vi "Read_raw_inst_setup.vi"(0 "Setup file":string) -> (8 "Setup string":string, 10 "Ch & spans choices":T4(array[cluster]) {"D" format="%.2f"; "Ch No" min=0; "low limit (-10V)" min=-10 max=10 format="%.2f"; "high limit (10V)" min=-10 max=10 format="%.2f"}, 13 "PWA Data":T1, 14 "Number of Analogue instruments":i32=1, 16 "LDA data":enum16{"No LDA data", "Take LDA data"}(ring)=enum."Take LDA data", 17 "LDA set up":T3={"dimensions"=enum."2D", "Analogue Freq Multiplier"=0.1} {"Analogue Freq Multiplier" min=0.1 max=100.0 format="%_5g"}, 19 "Synchronise Analogue channels with LDA":bool)   [LabVIEW 2014]
uses:
  Controls/Inst_type.ctl
  Controls/LDA_Setup.ctl
  Controls/PWA_Data.ctl
  Controls/Post_Process.ctl
  File/Setup_Filetype.ctl
  Controls/Trigger_Mode.ctl
  Controls/Tunnel_Coordinates.ctl
  Globals/Meas_global.vi
  Globals/LDA_meas_global_1.vi
  Globals/LDA_meas_global_2.vi
  Globals/Trav_pos_global.vi
panel:
  in  "Inst type":T2
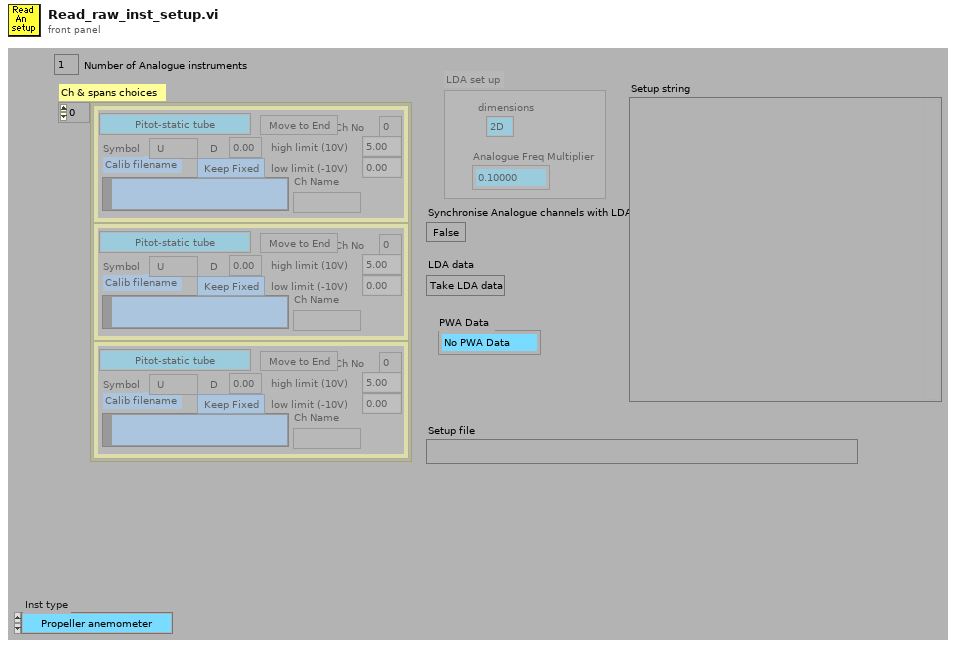
[diagram p1: front panel]
types:
  T1 = typedef "PWA_Data.ctl" = enum16{"No PWA Data", "One Ch PWA"}
  T2 = typedef "Inst_type.ctl" = enum16{"Propeller anemometer", "Raw voltage", "Pressure Transducer", "Pitot-static tube", "Preston tube", "Hot wire", "Cross wire 1", "Cross wire 2", "Generic Linear", "Generic Polynomial", "Generic BackPoly", "Fast FID", "Thermocouple", "Cold wire", "Pulsed Wire", "LDA Vel", "LDA Tran time", "LDA Arr time", "Microphone"}
  T3 = typedef "LDA_Setup.ctl" = cluster{"dimensions":enum16{"1D", "2D"}, "Analogue Freq Multiplier":dbl}
  T4 = cluster{"high limit (10V)":sgl, "low limit (-10V)":sgl, "Ch No":i16, "Calib filename":path, "Inst type":T2, "Symbol":string, "Move channel":bool, "Use Latest":bool, "D":dbl, "Ch Name":string}[]
  T5 = typedef "Post_Process.ctl" = enum16{"Take New Data", "Post Process Raw Data File"}
  T6 = typedef "Setup_Filetype.ctl" = enum16{"Measurement Setups", "Calibration Setups", "General", "Results File Plotter Setups", "Speed Calib Tweaks"}
  T7 = typedef "Trigger_Mode.ctl" = enum16{"Free Running", "Start on Trigger", "Trigger Every Block", "Trigger Every Sample"}
  T8 = typedef "Tunnel_Coordinates.ctl" = enum16{"Work in Tunnel Coordinates", "Work in Model Coordinates"}
  T9 = cluster{"high limit (10V)":sgl, "low limit (-10V)":sgl, "Ch No":i16, "Calib filename":path, "Inst type":T2, "Symbol":string, "Move channel":bool, "Use Latest":bool, "D":dbl, "Ch Name":string}
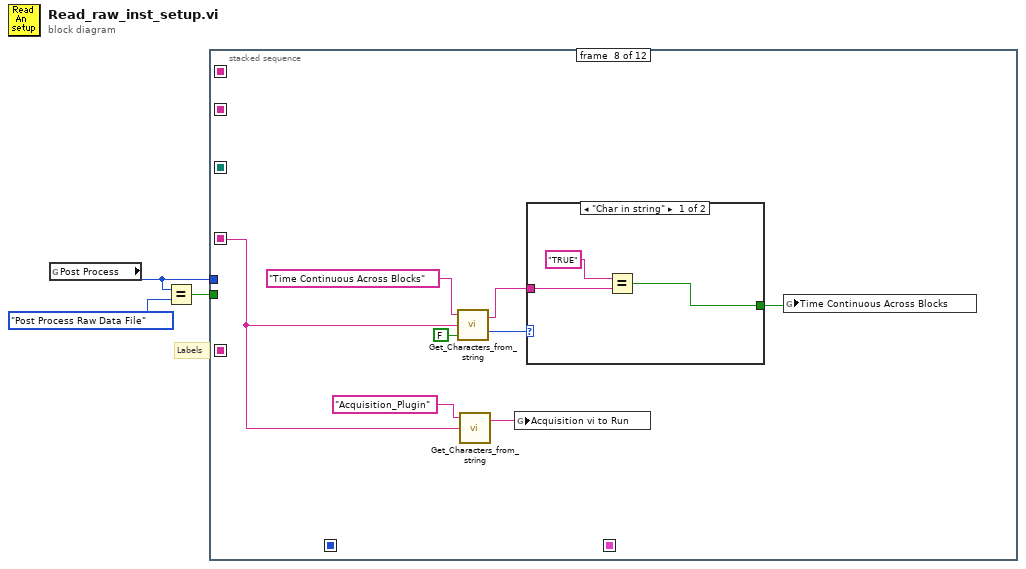
[diagram p0: block diagram]
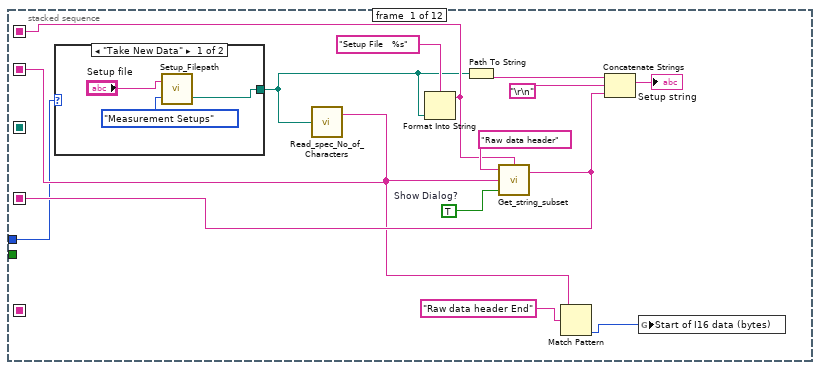
[diagram p2: hidden frame]
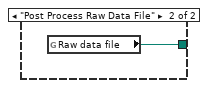
[diagram p3: hidden frame]
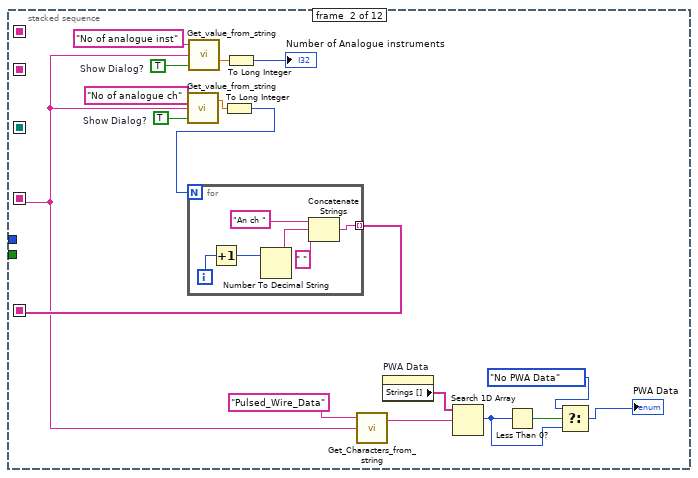
[diagram p4: hidden frame]
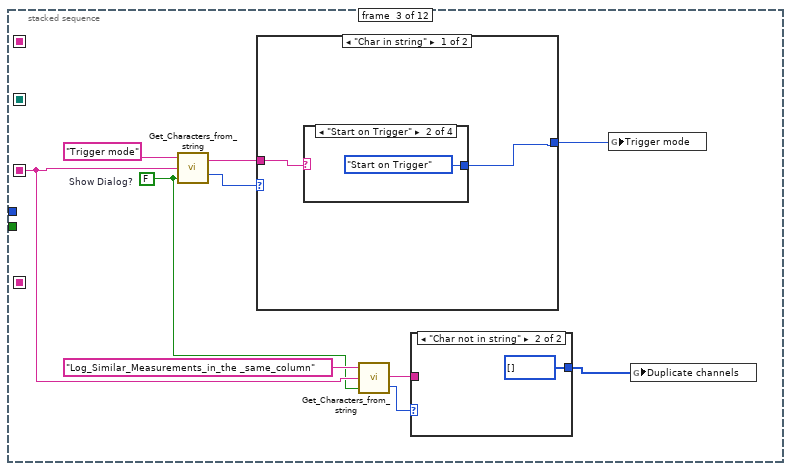
[diagram p5: hidden frame]
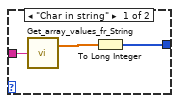
[diagram p6: hidden frame]
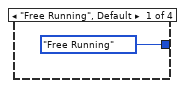
[diagram p7: hidden frame]
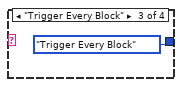
[diagram p8: hidden frame]
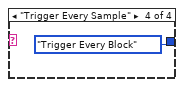
[diagram p9: hidden frame]
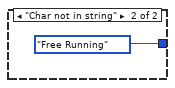
[diagram p10: hidden frame]
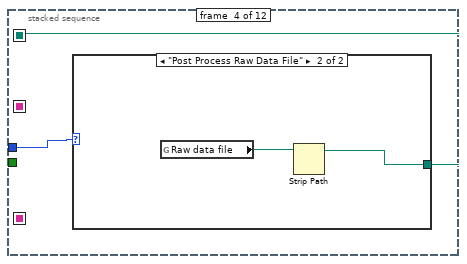
[diagram p11: hidden frame]
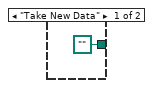
[diagram p12: hidden frame]
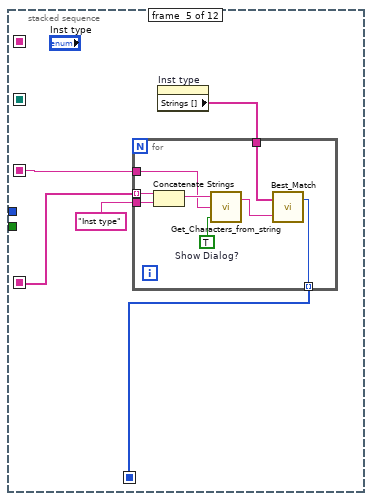
[diagram p13: hidden frame]
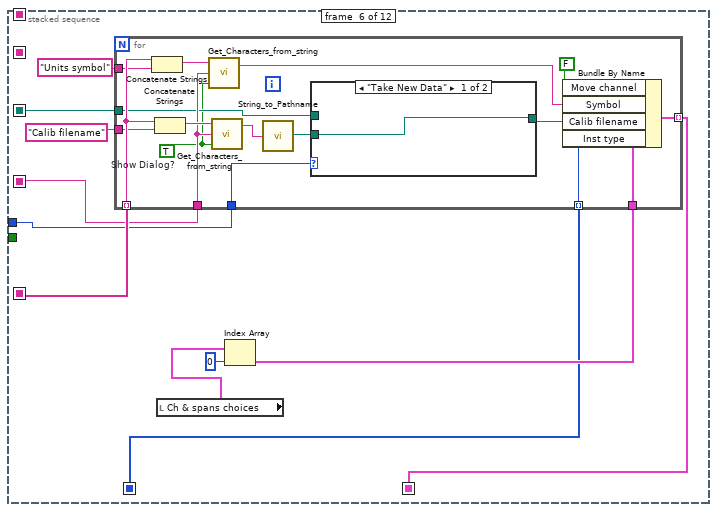
[diagram p14: hidden frame]
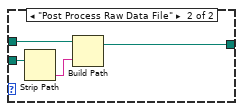
[diagram p15: hidden frame]
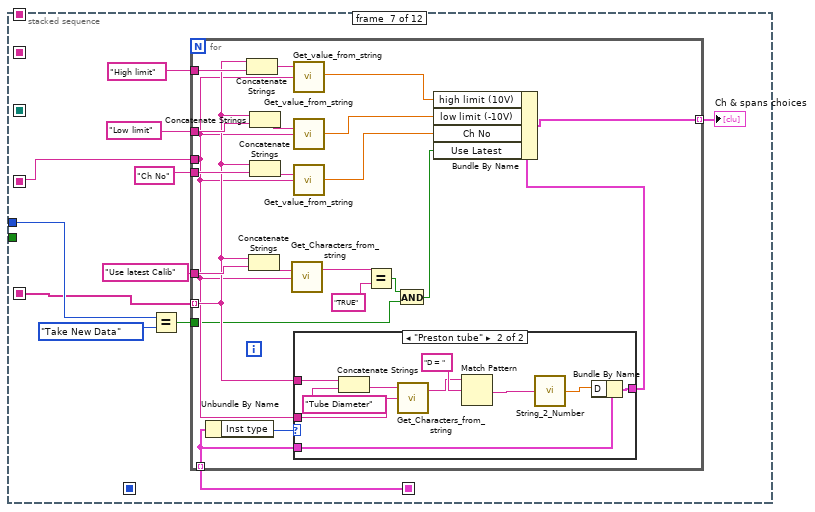
[diagram p16: hidden frame]
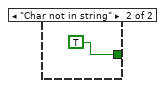
[diagram p18: hidden frame]
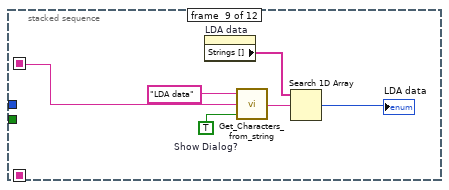
[diagram p19: hidden frame]
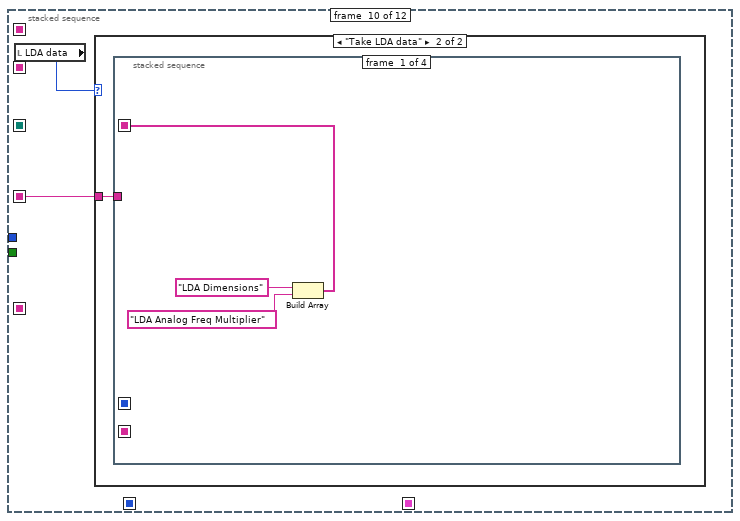
[diagram p20: hidden frame]
diagram:
  # "Labels"
  n1 = global read "Meas_global.vi" "Post Process"() -> (w1:T5)
  n2 = Equal?(x=w1, y=Post_Process."Post Process Raw Data File" ("Post Process")) -> (x = y?=w3:bool)
  n3 = stacked-sequence {
    seq-local: [w14 _ _ _ _ _ _ _ _ _ _ _] -> [_ w28 w48 _ w74 w84 w126 w165 w176 w179 w241 w265]
    seq-local: [_ w35 _ _ _ _ _ _ _ _ _ _] -> [_ _ _ _ w73 w93 w117 _ _ _ _ _]
    seq-local: [_ _ _ _ w70 _ _ _ _ _ _ _] -> [_ _ _ _ _ w87 _ _ _ _ _ _]
    seq-local: [_ _ _ _ _ w86 _ _ _ _ _ _] -> [_ _ _ _ _ _ w125 _ _ _ _ _]
    seq-local: [_ _ _ w66 _ _ _ _ _ _ _ _] -> [_ _ _ _ _ w85 _ _ _ _ _ _]
    seq-local: [w9 _ _ _ _ _ _ _ _ _ _ _] -> [_ _ _ _ _ _ _ _ _ _ _ w264]
    seq-local: [w6 _ _ _ _ _ _ _ _ _ _ _] -> [_ _ _ _ _ _ _ _ _ _ _ _]
    tunnel: w3 -> [_ _ _ _ _ _ _ _ _ _ _ w266]
    tunnel: w1 -> [w5 _ _ w65 _ w83 w118 _ _ _ _ _]
    frame #0 {
      w11 = TRUE  # Show Dialog?
      n4 = case shown="\"Take New Data\"" w5 {
        tunnel: [w17 w20] -> w4
        frame "Take New Data" {
          n5 = call "Setup_Filepath.vi"("Setup File Type"=Setup_Filetype."Measurement Setups", "Filename in"="Setup file") -> ("Filename Out"=w17:path)  [unwired: 1 out]
        }
        frame "Post Process Raw Data File" {
          n6 = global read "Meas_global.vi" "Raw data file"() -> (w20:path)
        }
      }
      n7 = call "Read_spec_No_of_Characters.vi"("Filename"=w4) -> ("character string"=w9:string)  [unwired: 1 out]
      n8 = Format Into String(format string="Setup File   %s", w4) -> (resulting string=w6:string)  [unwired: 2 in, 1 out]
      n9 = Path To String(path=w4) -> (string=w12:string)
      n10 = call "Get_string_subset.vi"("String Name"=w6, "Show Dialog?"=w11, "String to split"=w9, "File Label"="Raw data header") -> ("Output string"=w14:string)  [unwired: 1 out]
      n11 = Match Pattern(string=w9, regular expression="Raw data header End") -> (offset past match=w8:i32)  [unwired: 4 out]
      n12 = Concatenate Strings(w12, "\r\n", w14) -> (→"Setup string":string)
      n13 = global write "Meas_global.vi" "Start of I16 data (bytes)"(w8) -> ()
    }
    frame #1 {
      w29 = TRUE  # Show Dialog?
      w30 = TRUE  # Show Dialog?
      n14 = call "Get_value_from_string.vi"("Show Dialog?"=w30, "Input string"=w28, "Variable name"="No of analogue ch") -> ("Value"=w36:dbl)  [unwired: 1 out]
      n15 = call "Get_value_from_string.vi"("Show Dialog?"=w29, "Input string"=w28, "Variable name"="No of analogue inst") -> ("Value"=w33:dbl)  [unwired: 1 out]
      n16 = To Long Integer(number=w36) -> (32bit integer=w31:i32)
      n17 = for {
        N: w31 -> [_]
        tunnel: [w39] -> w35 mode=indexing
        i -> [w41]
        n18 = Increment(x=w41) -> (x+1=w40:i32)
        n19 = Number To Decimal String(number=w40) -> (decimal integer string=w43:string)  [unwired: 1 out]
        n20 = Concatenate Strings("An ch ", w43, " ") -> (w39:string)
      }
      n21 = To Long Integer(number=w33) -> (32bit integer=→"Number of Analogue instruments":i32)
      n22 = call "Get_Characters_from_string.vi"("Input string"=w28, "Variable name"="Pulsed_Wire_Data") -> ("Value"=w25:string)  [unwired: 1 in, 1 out]
      n23 = property on="PWA Data" class="Enum (strict)"() -> ("Strings []"=w26:string[])  [unwired: 2 in, 2 out]
      n24 = Search 1D Array(1D array=w26, element=w25) -> (index of element=w22:i32)  [unwired: 1 out]
      n25 = Less Than 0?(x=w22) -> (x < 0?=w24:bool)
      n26 = Select(t=PWA_Data."No PWA Data" ("PWA Data"), s=w24, f=w22) -> (s? t:f=→"PWA Data":i32)
    }
    frame #2 {
      w47 = FALSE  # Show Dialog?
      n27 = call "Get_Characters_from_string.vi"("Show Dialog?"=w47, "Input string"=w48, "Variable name"="Trigger mode") -> ("Status"=w52:enum16{"Char in string", "Char not in string"}, "Value"=w51:string)
      n28 = case shown="\"Char in string\"" w52 {
        tunnel: [w58 Trigger_Mode."Free Running" ("Trigger mode")] -> w50
        tunnel: w51 -> [w59 _]
        frame "Char in string" {
          n29 = case shown="\"Start on Trigger\"" w59 {
            tunnel: [Trigger_Mode."Free Running" ("Trigger mode") Trigger_Mode."Start on Trigger" ("Trigger mode") Trigger_Mode."Trigger Every Block" ("Trigger mode") Trigger_Mode."Trigger Every Block" ("Trigger mode")] -> w58
            frame "Free Running", Default {
            }
            frame "Start on Trigger" {
            }
            frame "Trigger Every Block" {
            }
            frame "Trigger Every Sample" {
            }
          }
        }
        frame "Char not in string" {
        }
      }
      n30 = call "Get_Characters_from_string.vi"("Show Dialog?"=w47, "Input string"=w48, "Variable name"="Log_Similar_Measurements_in_the _same_column") -> ("Status"=w44:enum16{"Char in string", "Char not in string"}, "Value"=w46:string)
      n31 = case shown="\"Char not in string\"" w44 {
        tunnel: w46 -> [w56 _]
        tunnel: [w54 i32[] []] -> w45
        frame "Char in string" {
          n32 = call "Get_array_values_fr_String.vi"("String Value"=w56) -> ("Numeric Array"=w55:dbl[])  [unwired: 1 out]
          n33 = To Long Integer(number=w55) -> (32bit integer=w54:i32[])
        }
        frame "Char not in string" {
        }
      }
      n34 = global write "Meas_global.vi" "Trigger mode"(w50) -> ()
      n35 = global write "Meas_global.vi" "Duplicate channels"(w45) -> ()
    }
    frame #3 {
      n36 = case shown="\"Post Process Raw Data File\"" w65 {
        tunnel: [path "" ("stripped path") w68] -> w66
        frame "Take New Data" {
        }
        frame "Post Process Raw Data File" {
          n37 = global read "Meas_global.vi" "Raw data file"() -> (w69:path)
          n38 = Strip Path(path=w69) -> (stripped path=w68:path)  [unwired: 1 out]
        }
      }
    }
    frame #4 {
      n39 = property on="Inst type" class="Enum (strict)"() -> ("Strings []"=w71:string[])  [unwired: 2 in, 2 out]
      n40 = for {
        tunnel: w74 -> [w81]
        tunnel: w71 -> [w77]
        tunnel: w73 -> [w80] mode=indexing
        tunnel: "Inst type" -> [w79]
        tunnel: [w75] -> w70 mode=indexing
        w78 = TRUE  # Show Dialog?
        n41 = Concatenate Strings(w80, w79) -> (w82:string)
        n42 = call "Get_Characters_from_string.vi"("Show Dialog?"=w78, "Input string"=w81, "Variable name"=w82) -> ("Value"=w76:string)  [unwired: 1 out]
        n43 = call "Best_Match.vi"("Input String"=w76, "String Options"=w77) -> ("index of element"=w75:i32)  [unwired: 1 out]
      }
    }
    frame #5 {
      n44 = local read "Ch & spans choices"() -> (w89:T4)
      n45 = Index Array(array=w89, index=0) -> (element=w88:T9)
      n46 = for {
        tunnel: w93 -> [w108] mode=indexing
        tunnel: "Calib filename" -> [w107]
        tunnel: "Units symbol" -> [w106]
        tunnel: w88 -> [w105]
        tunnel: w87 -> [w103] mode=indexing
        tunnel: [w102] -> w86 mode=indexing
        tunnel: w84 -> [w101]
        tunnel: w83 -> [w100]
        tunnel: w85 -> [w99]
        w96 = TRUE  # Show Dialog?
        n47 = Concatenate Strings(w108, w106) -> (w110:string)
        n48 = Concatenate Strings(w108, w107) -> (w109:string)
        n49 = call "Get_Characters_from_string.vi"("Show Dialog?"=w96, "Input string"=w101, "Variable name"=w110) -> ("Value"=w104:string)  [unwired: 1 out]
        n50 = call "Get_Characters_from_string.vi"("Show Dialog?"=w96, "Input string"=w101, "Variable name"=w109) -> ("Value"=w95:string)  [unwired: 1 out]
        n51 = call "String_to_Pathname.vi"("Input String"=w95) -> ("path"=w94:path)
        n52 = case shown="\"Take New Data\"" w100 {
          tunnel: w94 -> [w111 w115]
          tunnel: w99 -> [_ w112]
          tunnel: [w111 w113] -> w98
          frame "Take New Data" {
          }
          frame "Post Process Raw Data File" {
            n53 = Strip Path(path=w115) -> (name=w114:string)  [unwired: 1 out]
            n54 = Build Path(base path=w112, name or relative path=w114) -> (appended path=w113:path)
          }
        }
        n55 = Bundle By Name(cluster=w105, "Move channel"=FALSE, "Symbol"=w104, "Calib filename"=w98, "Inst type"=w103) -> (w102:T9)
      }
    }
    frame #6 {
      n56 = Equal?(x=w118, y=Post_Process."Take New Data" ("Post Process")) -> (x = y?=w116:bool)
      n57 = for {
        tunnel: "Low limit" -> [w148]
        tunnel: "High limit" -> [w147]
        tunnel: w125 -> [w129] mode=indexing
        tunnel: [w139] -> w124 mode=indexing
        tunnel: w126 -> [w131]
        tunnel: "Ch No" -> [w143]
        tunnel: "Use latest Calib" -> [w137]
        tunnel: w117 -> [w132] mode=indexing
        tunnel: w116 -> [w130]
        n58 = Unbundle By Name(w129) -> ("Inst type"=w133:T2)
        n59 = Concatenate Strings(w132, w147) -> (w146:string)
        n60 = Concatenate Strings(w132, w137) -> (w138:string)
        n61 = Concatenate Strings(w132, w148) -> (w145:string)
        n62 = Concatenate Strings(w132, w143) -> (w144:string)
        n63 = call "Get_Characters_from_string.vi"("Input string"=w131, "Variable name"=w138) -> ("Value"=w136:string)  [unwired: 1 in, 1 out]
        n64 = call "Get_value_from_string.vi"("Input string"=w131, "Variable name"=w146) -> ("Value"=w142:dbl)  [unwired: 1 in, 1 out]
        n65 = call "Get_value_from_string.vi"("Input string"=w131, "Variable name"=w145) -> ("Value"=w141:dbl)  [unwired: 1 in, 1 out]
        n66 = call "Get_value_from_string.vi"("Input string"=w131, "Variable name"=w144) -> ("Value"=w140:dbl)  [unwired: 1 in, 1 out]
        n67 = case shown="\"Preston tube\"" w133 {
          tunnel: w132 -> [_ w159]
          tunnel: w131 -> [_ w154]
          tunnel: w129 -> [w149 w157]
          tunnel: [w149 w156] -> w128
          frame "Propeller anemometer", Default {
          }
          frame "Preston tube" {
            n68 = Concatenate Strings(w159, "Tube Diameter") -> (w155:string)
            n69 = call "Get_Characters_from_string.vi"("Input string"=w154, "Variable name"=w155) -> ("Value"=w152:string)  [unwired: 1 in, 1 out]
            n70 = Match Pattern(string=w152, regular expression="D = " ("String to match")) -> (after substring=w151:string)  [unwired: 4 out]
            n71 = call "String_2_Number.vi"("Value"=w151) -> ("Numeric"=w150:dbl)
            n72 = Bundle By Name(cluster=w157, "D"=w150) -> (w156:T9)
          }
        }
        n73 = Equal?(x=w136, y="TRUE") -> (x = y?=w134:bool)
        n74 = And(x=w134, y=w130) -> (x .and. y?=w127:bool)
        n75 = Bundle By Name(cluster=w128, "high limit (10V)"=w142, "low limit (-10V)"=w141, "Ch No"=w140, "Use Latest"=w127) -> (w139:T9)
      }
      "Ch & spans choices" <- w124
    }
    frame #7 {
      n76 = call "Get_Characters_from_string.vi"("Show Dialog?"=FALSE, "Input string"=w165, "Variable name"="Time Continuous Across Blocks") -> ("Status"=w162:enum16{"Char in string", "Char not in string"}, "Value"=w160:string)
      n77 = call "Get_Characters_from_string.vi"("Input string"=w165, "Variable name"="Acquisition_Plugin") -> ("Value"=w166:string)  [unwired: 1 in, 1 out]
      n78 = global write "Meas_global.vi" "Acquisition vi to Run"(w166) -> ()
      n79 = case shown="\"Char in string\"" w162 {
        tunnel: [w168 TRUE ("Time Continuous Across Blocks")] -> w161
        tunnel: w160 -> [w170 _]
        frame "Char in string" {
          n80 = Equal?(x="TRUE", y=w170) -> (x = y?=w168:bool)
        }
        frame "Char not in string" {
        }
      }
      n81 = global write "Meas_global.vi" "Time Continuous Across Blocks"(w161) -> ()
    }
    frame #8 {
      w173 = TRUE  # Show Dialog?
      n82 = property on="LDA data" class="Enum (strict)"() -> ("Strings []"=w172:string[])  [unwired: 2 in, 2 out]
      n83 = call "Get_Characters_from_string.vi"("Show Dialog?"=w173, "Input string"=w176, "Variable name"="LDA data" ("Label for characters")) -> ("Value"=w177:string)  [unwired: 1 out]
      n84 = Search 1D Array(1D array=w172, element=w177) -> (index of element=→"LDA data":i32)  [unwired: 1 out]
    }
    frame #9 {
      n85 = local read "LDA data"() -> (w178:enum16{"No LDA data", "Take LDA data"})
      n86 = case shown="\"Take LDA data\"" w178 {
        tunnel: w179 -> [_ w180]
        frame "No LDA data" {
        }
        frame "Take LDA data" {
          n87 = stacked-sequence {
            seq-local: [_ w186 _ _] -> [_ _ w212 _]
            seq-local: [_ _ w211 _] -> [_ _ _ w222]
            seq-local: [w182 _ _ _] -> [_ w188 _ _]
            tunnel: w180 -> [_ w185 _ w223]
            frame #0 {
              n88 = Build Array("LDA Dimensions", "LDA Analog Freq Multiplier") -> (w182:string[])
            }
            frame #1 {
              n89 = local read "LDA set up"() -> (w187:T3)
              n90 = for {
                tunnel: w188 -> [w194] mode=indexing
                shift-right: [w191] -> w184
                shift-left: w187 -> [w192]
                tunnel: w185 -> [w189]
                n91 = call "Get_Characters_from_string.vi"("Input string"=w189, "Variable name"=w194) -> ("Status"=w193:enum16{"Char in string", "Char not in string"}, "Value"=w190:string)  [unwired: 1 in]
                n92 = case shown="\"Char in string\"" w193 {
                  tunnel: w194 -> [w198 _]
                  tunnel: w192 -> [w197 w210]
                  tunnel: [w196 w210] -> w191
                  tunnel: w190 -> [w195 _]
                  frame "Char in string" {
                    n93 = case shown="\"LDA Analog Freq Multiplier\"" w198 {
                      tunnel: w197 -> [w202 w208 w209]
                      tunnel: [w201 w207 w209] -> w196
                      tunnel: w195 -> [w200 w206 _]
                      frame "LDA Dimensions" {
                        n94 = case shown="\"2D\", Default" w200 {
                          tunnel: [enum16{"1D", "2D"}."1D" ("Bundle Element") enum16{"1D", "2D"}."2D" ("Bundle Element")] -> w199
                          frame "1D" {
                          }
                          frame "2D", Default {
                          }
                        }
                        n95 = Bundle By Name(cluster=w202, "dimensions"=w199) -> (w201:T3)
                      }
                      frame "LDA Analog Freq Multiplier" {
                        n96 = Fract/Exp String To Number(string=w206) -> (number=w205:dbl)  [unwired: 3 in, 1 out]
                        n97 = Bundle By Name(cluster=w208, "Analogue Freq Multiplier"=w205) -> (w207:T3)
                      }
                      frame "No Match", Default {
                      }
                    }
                  }
                  frame "Char not in string" {
                  }
                }
              }
              "LDA set up" <- w184
              n98 = Unbundle By Name(w184) -> ("dimensions"=w186:enum16{"1D", "2D"})
            }
            frame #2 {
              n99 = case shown="\"1D\"" w212 {
                tunnel: [1 2] -> w213
                frame "1D" {
                }
                frame "2D" {
                }
              }
              n100 = for {
                N: w213 -> [_]
                tunnel: [w215] -> w211 mode=indexing
                i -> [w217]
                n101 = Increment(x=w217) -> (x+1=w216:i32)
                n102 = Number To Decimal String(number=w216) -> (decimal integer string=w219:string)  [unwired: 1 out]
                n103 = Concatenate Strings("BSA ", w219, " ") -> (w215:string)
              }
            }
            frame #3 {
              n104 = for {
                tunnel: w223 -> [w225]
                tunnel: w222 -> [w226] mode=indexing
                i -> [w235]
                n105 = Concatenate Strings(w226, "Component") -> (w236:string)
                n106 = Concatenate Strings(w226, "Multiply Velocity by -1") -> (w230:string)
                n107 = Increment(x=w235) -> (x+1=w232:i32)
                n108 = call "Get_Characters_from_string.vi"("Input string"=w225, "Variable name"=w236) -> ("Value"=w233:string)  [unwired: 1 in, 1 out]
                n109 = call "Get_Characters_from_string.vi"("Show Dialog?"=FALSE, "Input string"=w225, "Variable name"=w230) -> ("Value"=w228:string)  [unwired: 1 out]
                n110 = Equal?(x=w228, y="TRUE") -> (x = y?=w224:bool)
                n111 = case shown="2" w232 {
                  tunnel: w233 -> [w238 w240]
                  tunnel: w224 -> [w237 w239]
                  frame 1, Default {
                    n112 = global write "LDA_meas_global_1.vi" "Vel Comp BSA1"(w238) -> ()
                    n113 = global write "LDA_meas_global_1.vi" "Multiply Velocity by -1"(w237) -> ()
                  }
                  frame 2 {
                    n114 = global write "LDA_meas_global_2.vi" "Vel Comp BSA2"(w240) -> ()
                    n115 = global write "LDA_meas_global_2.vi" "Multiply Velocity by -1"(w239) -> ()
                  }
                }
              }
            }
          }
        }
      }
    }
    frame #10 {
      n116 = Build Array("Synchronise with LDA") -> (w251:string[])
      n117 = Build Array("FALSE", "TRUE") -> (w248:string[])
      n118 = call "Get_value_from_string.vi"("Input string"=w241, "Variable name"="Sync Delay Time (ms)" ("Label for characters")) -> ("Status"=w243:enum16{"Char in string", "Char not in string"}, "Value"=w242:dbl)  [unwired: 1 in]
      n119 = case shown="\"Char in string\"" w243 {
        tunnel: w242 -> [w253 _]
        frame "Char in string" {
          n120 = global write "LDA_meas_global_1.vi" "Sync Delay Time (ms)"(w253) -> ()
        }
        frame "Char not in string" {
        }
      }
      n121 = Build Array(FALSE, TRUE) -> (w245:bool[])
      n122 = for {
        tunnel: w241 -> [w261]
        tunnel: w251 -> [w257] mode=indexing
        tunnel: w248 -> [w256]
        tunnel: w245 -> [w255]
        i -> [w259]
        w254 = TRUE  # Show Dialog?
        n123 = call "Get_Characters_from_string.vi"("Show Dialog?"=w254, "Input string"=w261, "Variable name"=w257) -> ("Value"=w262:string)  [unwired: 1 out]
        n124 = Search 1D Array(1D array=w256, element=w262) -> (index of element=w260:i32)  [unwired: 1 out]
        n125 = Index Array(array=w255, index=w260) -> (element=w258:bool)
        n126 = case shown="1" w259 {
          tunnel: w258 -> [w263 _]
          frame 0, Default {
            "Synchronise Analogue channels with LDA" <- w263
          }
          frame 1 {
          }
        }
      }
    }
    frame #11 {
      n127 = case shown="True" w266 {
        tunnel: w265 -> [_ w272]
        tunnel: w264 -> [_ w267]
        frame False {
        }
        frame True {
          w271 = FALSE  # Show Dialog?
          n128 = call "Get_Characters_from_string.vi"("Show Dialog?"=w271, "Input string"=w272, "Variable name"="Coordinate_System" ("Label for characters")) -> ("Status"=w270:enum16{"Char in string", "Char not in string"}, "Value"=w269:string)
          n129 = case shown="\"Char not in string\"" w270 {
            tunnel: w269 -> [w275 _]
            tunnel: [w274 w278] -> w268
            tunnel: w267 -> [_ w280]
            frame "Char in string" {
              n130 = case shown="\"Work in Model Coordinates\"" w275 {
                tunnel: [Tunnel_Coordinates."Work in Model Coordinates" ("Work in Tunnel Coordinates?") Tunnel_Coordinates."Work in Tunnel Coordinates" ("Work in Tunnel Coordinates?")] -> w274
                frame "Work in Model Coordinates" {
                }
                frame "Work in Tunnel Coordinates", Default {
                }
              }
            }
            frame "Char not in string" {
              n131 = Concatenate Strings("X Pos (Model)", "\t", "Y Pos (Model)") -> (w281:string)
              n132 = Match Pattern(string=w280, regular expression=w281) -> (offset past match=w279:i32)  [unwired: 4 out]
              n133 = case shown="-1" w279 {
                tunnel: [Tunnel_Coordinates."Work in Model Coordinates" ("Work in Tunnel Coordinates?") Tunnel_Coordinates."Work in Tunnel Coordinates" ("Work in Tunnel Coordinates?")] -> w278
                frame 0, Default {
                }
                frame -1 {
                }
              }
            }
          }
          n134 = global write "Trav_pos_global.vi" "Work in Tunnel Coordinates?"(w268) -> ()
        }
      }
    }
  }
